vi "Create PPL.vi"(0 "Project Refnum":refnum<vi>, 5 "Plug-in name":string, 11 "error in (no error)":errorcluster) -> (4 "project ref out":refnum<vi>, 6 "path":path, 15 "error out":errorcluster)   [LabVIEW 2021, in "NI_AB_API_PPL_Extensions.lvclass"]
uses:
  NI_AB_API_PPL_Extensions.lvclass
  NI_AB_API_PPL_Extensions.lvclass/NI_AB_API_PPL_Extensions.ctl
  InstrumentStudio Plug-In Editor.lvlib
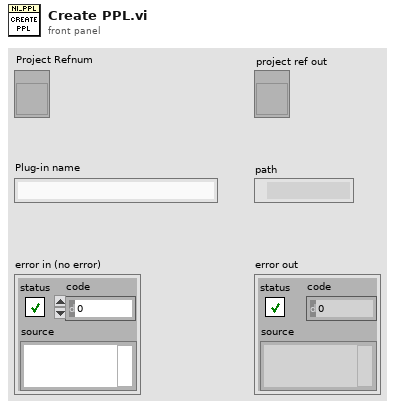
[diagram p1: front panel]
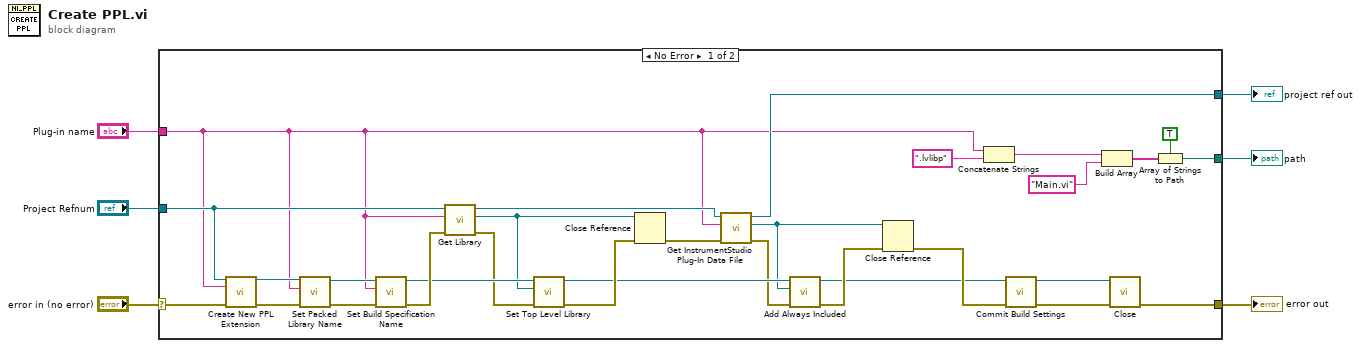
[diagram p0: block diagram]
diagram:
  n1 = case shown="No Error" "error in (no error)" {
    selector: "error in (no error)" -> [w36 w38]
    tunnel: [w7 w38] -> w1
    tunnel: "Project Refnum" -> [w35 w37]
    tunnel: "Plug-in name" -> [w16 _]
    tunnel: [w17 w37] -> w3
    tunnel: [w23 _] -> w2
    frame No Error {
      n2 = call "Create New PPL Extension.vi"("Project Refnum"=w35, "Build specification name"=w16, "error in (no error)"=w36) -> ("NI_AB_API_Build out"=w22:refnum<class "NI_AB_API_PPL_Extensions.lvclass">, "error out"=w19:errorcluster)  [unwired: 11 in]
      n3 = call-dynamic "Set Packed Library Name.vi"("error in (no error)"=w19, "Packed library name"=w16, "PPL in"=w22) -> ("error out"=w20:errorcluster, "PPL out"=w21:refnum<class "NI_AB_API_PPL_Extensions.lvclass">)  [unwired: 7 in]
      n4 = call-dynamic "Set Build Specification Name.vi"("error in (no error)"=w20, "Build Specification Name"=w16, "NI_AB_API_PPL in"=w21) -> ("error out"=w34:errorcluster, "NI_AB_API_PPL out"=w33:refnum<class "NI_AB_API_PPL_Extensions.lvclass">)  [unwired: 7 in]
      n5 = call "Get Library.vi"("error in"=w34, "library name"=w16, "project ref"=w35) -> ("error out"=w32:errorcluster, "library item"=w26:refnum<vi>, "project ref out"=w18:refnum<vi>)  [unwired: 5 in, 1 out]
      n6 = call-dynamic "Set Top Level Library.vi"("error in (no error)"=w32, "ProjectItem Refnum"=w26, "PPL in"=w33) -> ("error out"=w30:errorcluster, "PPL out"=w15:refnum<class "NI_AB_API_PPL_Extensions.lvclass">)  [unwired: 7 in]
      n7 = Close Reference(reference=w26, error in (no error)=w30) -> (error out=w9:errorcluster)
      n8 = call "Get InstrumentStudio Plug-In Data File.vi"("error in"=w9, "library name"=w16, "project ref"=w18) -> ("error out"=w10:errorcluster, "Document item"=w14:refnum<vi>, "project ref out"=w17:refnum<vi>)  [unwired: 5 in, 1 out]
      n9 = call-dynamic "Add Always Included.vi"("error in (no error)"=w10, "ProjectItem Refnum"=w14, "PPL in"=w15) -> ("error out"=w13:errorcluster, "PPL out"=w11:refnum<class "NI_AB_API_PPL_Extensions.lvclass">)  [unwired: 7 in]
      n10 = Close Reference(reference=w14, error in (no error)=w13) -> (error out=w12:errorcluster)
      n11 = Concatenate Strings(w16, ".lvlibp" ("string")) -> (w28:string)
      n12 = call-dynamic "Commit Build Settings.vi"("error in (no error)"=w12, "PPL in"=w11) -> ("error out"=w31:errorcluster, "PPL out"=w27:refnum<class "NI_AB_API_PPL_Extensions.lvclass">)  [unwired: 8 in]
      n13 = Build Array(w28, "Main.vi" ("element")) -> (w24:string[])
      n14 = call-dynamic "Close.vi"("error in (no error)"=w31, "DLL in"=w27) -> ("error out"=w7:errorcluster)  [unwired: 9 in]
      n15 = Array of Strings to Path(0:w24, 1:TRUE ("relative")) -> (2:w23:path)
    }
    frame Error {
    }
  }
  "error out" <- w1
  "project ref out" <- w3
  "path" <- w2
